vi "Fuzzy2Drone.vi"() -> ()   [LabVIEW 2014]
uses:
  <vilib>/LVH/AR Drone Toolkit/Decode NavData/Typedefs/NavData Demo.ctl
  <vilib>/LVH/AR Drone Toolkit/AR Drone.lvlib
panel:
  in  "Vertical Pointer Slide":u8(slide) scale=0.0..220.0
  in  "YawPosition":i16(knob) scale=-180.0..180.0
  out "NavData Out":T1
  out "Battery Remaining":dbl(slide) scale=0.0..100.0
  in  "stop":bool
  out "Axes Output":T2 {"Vertical Speed" scale=-1.0..1.0; "Yaw Speed" scale=-1.0..1.0; "Pitch" scale=-1.0..1.0; "Roll" scale=-1.0..1.0}
  out "Gamepad Output":T3
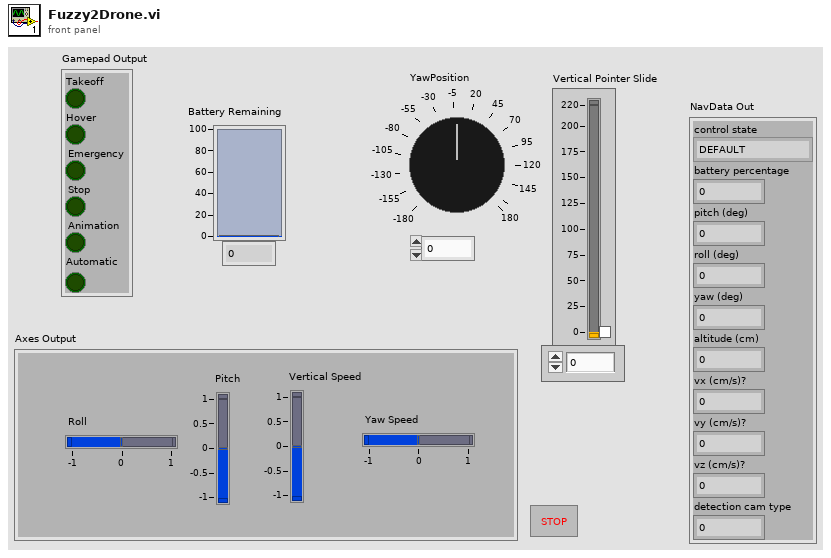
[diagram p1: front panel]
types:
  T1 = typedef "AR Drone.lvlib/NavData Demo.ctl" = cluster{"control state":enum32{"DEFAULT", "INIT", "LANDING", "FLYING", "HOVERING", "TEST", "TRANS_TAKEOFF", "TRANS_GOTOFIX", "TRANS_LANDING"}, "battery percentage":u32, "pitch (deg)":sgl, "roll (deg)":sgl, "yaw (deg)":sgl, "altitude (cm)":u32, "vx (cm/s)?":sgl, "vy (cm/s)?":sgl, "vz (cm/s)?":sgl, "detection cam type":u32}
  T2 = cluster{"Roll":dbl, "Pitch":dbl, "Vertical Speed":dbl, "Yaw Speed":dbl}
  T3 = cluster{"Takeoff":bool, "Hover":bool, "Emergency":bool, "Stop":bool, "Animation":bool, "Automatic":bool}
  T4 = typedef "AR Drone.lvlib/AR Drone Resource.ctl" = cluster{"UDP Control Connection":refnum<k16>, "UDP NavData Connection":refnum<k16>, "UDP Video Connection (Drone 1.0)":refnum<k16>, "TCP Video Connection (Drone 2.0)":refnum<k5>, "TCP Control Port Connection":refnum<k5>, "Drone IP address":string, "Drone Command Port":u16, "Drone NavData Port":u16, "Drone Vid Stream Port":u16, "Drone TCP Control Port":u16, "Home IP address":string, "Home Command Port":u16, "Home NavData Port":u16, "Home Vid Stream Port":u16, "Drone Version":i32}
  T5 = cluster{"Roll":sgl, "Pitch":sgl, "Vertical Speed":sgl, "Yaw Speed":sgl}
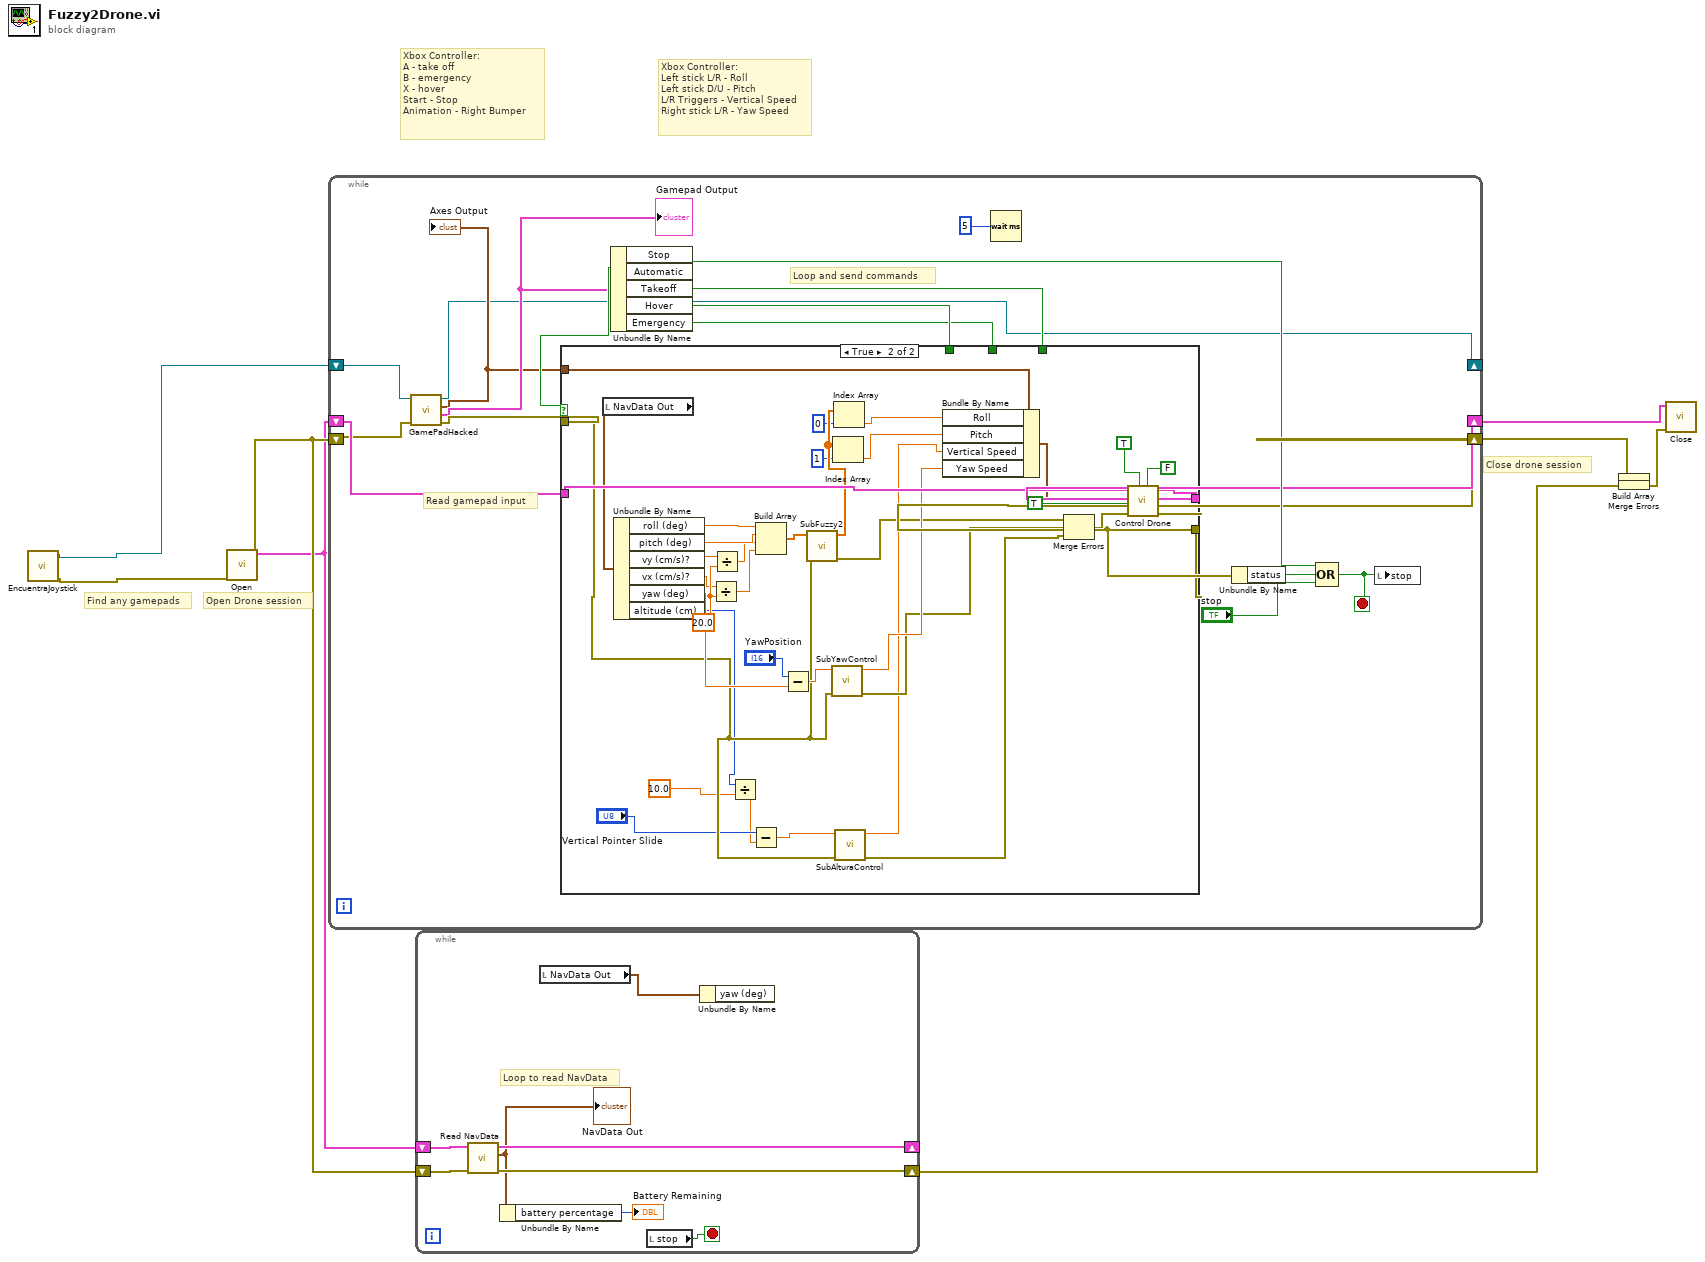
[diagram p0: block diagram]
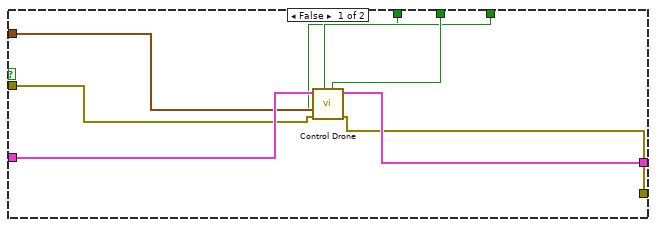
[diagram p2: hidden frame]
diagram:
  # "Close drone session"
  # "Open Drone session"
  # "Find any gamepads"
  # "Xbox Controller:\nLeft stick L/R - Roll\nLeft stick D/U - Pitch\nL/R Triggers - Vertical Speed\nRight stick L/R - Yaw Speed"
  # "Xbox Controller:\nA - take off\nB - emergency\nX - hover\nStart - Stop\nAnimation - Right Bumper"
  n1 = call "EncuentraJoystick.vi"() -> ("error out"=w2:errorcluster, "Refnum out"=w3:refnum<k1>)  [unwired: 10 in]
  n2 = call <vilib>:"Open.vi"("error in (no error)"=w2) -> ("error out"=w6:errorcluster, "AR Drone Resource"=w4:T4)  [unwired: 9 in]
  n3 = while {
    shift-right: [w20] -> w1
    shift-left: w4 -> [w21]
    shift-right: [w19] -> w8
    shift-left: w6 -> [w14]
    shift-right: [w10] -> _
    shift-left: w3 -> [w15]
    stop <- w25 stop-if-true
    # "Loop and send commands"
    # "Read gamepad input"
    n4 = call "GamePadHacked.vi"("error in (no error)"=w14, "Refnum in"=w15) -> ("error out"=w13:errorcluster, "Gamepad Output"=w12:T3, "Control Cluster"=w11:T5, "Refnum out"=w10:refnum<k1>)  [unwired: 6 in]
    "Axes Output" <- w11
    "Gamepad Output" <- w12
    n5 = Unbundle By Name(w12) -> ("Stop"=w22:bool, "Automatic"=w23:bool, "Takeoff"=w18:bool, "Hover"=w17:bool, "Emergency"=w16:bool)
    n6 = case shown="True" w23 {
      tunnel: [w33 w71] -> w19
      tunnel: w21 -> [w34 w72]
      tunnel: [w35 w70] -> w20
      tunnel: w18 -> [w30 _]
      tunnel: w17 -> [w29 _]
      tunnel: w16 -> [w31 _]
      tunnel: w11 -> [w32 w36]
      tunnel: w13 -> [w28 w45]
      frame False {
        n7 = call <vilib>:"Control Drone.vi"("Emergency Landing"=w31, "Takeoff/Land"=w30, "error in (no error)"=w28, "Hover"=w29, "Control Cluster"=w32, "AR Drone Resource"=w34) -> ("error out"=w33:errorcluster, "AR Drone Resource Out"=w35:T4)  [unwired: 4 in]
      }
      frame True {
        w54 = 20.0 ("y")
        n8 = local read "NavData Out"() -> (w67:T1)
        n9 = Unbundle By Name(w67) -> ("roll (deg)"=w64:sgl, "pitch (deg)"=w63:sgl, "vy (cm/s)?"=w52:sgl, "vx (cm/s)?"=w53:sgl, "yaw (deg)"=w49:sgl, "altitude (cm)"=w37:u32)
        n10 = Divide(x=w53, y=w54) -> (x/y=w55:dbl)
        n11 = Divide(x=w52, y=w54) -> (x/y=w56:dbl)
        n12 = Divide(x=w37, y=10.0) -> (x/y=w39:dbl)
        n13 = Subtract(x="Vertical Pointer Slide", y=w39) -> (x-y=w44:dbl)
        n14 = Build Array(w64, w63, w56, w55) -> (w57:dbl[])
        n15 = Subtract(x="YawPosition", y=w49) -> (x-y=w51:sgl)
        n16 = call "SubFuzzy2.vi"("error in (no error)"=w45, "input values"=w57) -> ("error out"=w46:errorcluster, "output values"=w60:dbl[])  [unwired: 8 in]
        n17 = call "SubYawControl.vi"("error in (no error)"=w45, "input value"=w51) -> ("error out"=w47:errorcluster, "output value"=w48:dbl)  [unwired: 8 in]
        n18 = Index Array(array=w60, index=1) -> (element=w61:dbl)
        n19 = Index Array(array=w60, index=0) -> (element=w62:dbl)
        n20 = call "SubAlturaControl.vi"("error in (no error)"=w45, "input value"=w44) -> ("error out"=w41:errorcluster, "output value"=w42:dbl)  [unwired: 8 in]
        n21 = Bundle By Name(cluster=w36, "Roll"=w62, "Pitch"=w61, "Vertical Speed"=w42, "Yaw Speed"=w48) -> (w66:T5)
        n22 = Merge Errors(w46, w47, w41) -> (w43:errorcluster)
        n23 = call <vilib>:"Control Drone.vi"("Emergency Landing"=FALSE, "Takeoff/Land"=TRUE, "error in (no error)"=w43, "Hover"=TRUE, "Control Cluster"=w66, "AR Drone Resource"=w72) -> ("error out"=w71:errorcluster, "AR Drone Resource Out"=w70:T4)  [unwired: 4 in]
      }
    }
    n24 = Wait (ms)(milliseconds to wait=u32 5) -> ()  [unwired: 1 out]
    n25 = Unbundle By Name(w19) -> ("status"=w24:bool)
    n26 = Compound Arithmetic op=OR(w22, w24, "stop") -> (w25:bool)
    n27 = local write "stop"(w25) -> ()
  }
  n28 = while {
    shift-right: [w79] -> _
    shift-left: w4 -> [w80]
    shift-right: [w77] -> w7
    shift-left: w6 -> [w78]
    stop <- w74 stop-if-true
    # "Loop to read NavData"
    n29 = call <vilib>:"Read NavData.vi"("error in (no error)"=w78, "AR Drone Resource"=w80) -> ("error out"=w77:errorcluster, "NavData Out"=w76:T1, "AR Drone Resource Out"=w79:T4)  [unwired: 7 in]
    "NavData Out" <- w76
    n30 = Unbundle By Name(w76) -> ("battery percentage"=→"Battery Remaining":u32)
    n31 = local read "NavData Out"() -> (w73:T1)
    n32 = local read "stop"() -> (w74:bool)
    n33 = Unbundle By Name(w73) -> ()  [unwired: 1 out]
  }
  n34 = Build Array(w8, w7) -> (w5:errorcluster[])
  n35 = Merge Errors(w5) -> (w9:errorcluster)
  n36 = call <vilib>:"Close.vi"("error in (no error)"=w9, "AR Drone Resource"=w1) -> ()  [unwired: 9 in, 1 out]
